vi "Init Package.vi"(7 "Logger":refnum<class "Logger.lvclass">, 8 "error in (no error)":errorcluster, 11 "GPackCLI in":refnum<class "GPackCLI.lvclass">) -> (0 "error out":errorcluster, 3 "GPackCLI out":refnum<class "GPackCLI.lvclass">)   [LabVIEW 2020, in "GPackTools.lvlib" / "GPackCLI.lvclass"]
uses:
  GPackCLI.lvclass
  GPack/Logger/Logger.lvclass
  GPackCLI.lvclass/GPackCLI.ctl
  CLIAction/CLIAction.lvclass
  GPack/PackageAbstract/PackageAbstract.lvclass
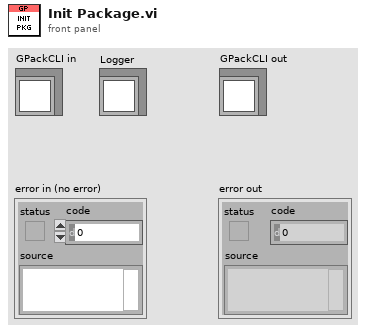
[diagram p1: front panel]
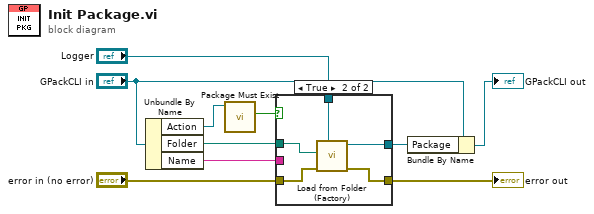
[diagram p0: block diagram]
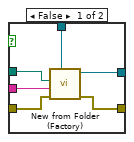
[diagram p2: hidden frame]
diagram:
  n1 = Unbundle By Name("GPackCLI in") -> ("Action"=w3:refnum<class "CLIAction.lvclass">, "Folder"=w9:path, "Name"=w6:string)
  n2 = call-dynamic "Package Must Exist.vi"("CLIAction in"=w3) -> ("Pkg Must Exist"=w2:bool)  [unwired: 8 in, 2 out]
  n3 = case shown="True" w2 {
    tunnel: w9 -> [w16 w21]
    tunnel: [w15 w20] -> w7
    tunnel: w6 -> [w14 _]
    tunnel: "error in (no error)" -> [w13 w19]
    tunnel: [w12 w18] -> w4
    tunnel: "Logger" -> [w11 w17]
    frame False {
      n4 = call "New from Folder (Factory).vi"("Logger"=w11, "error in (no error)"=w13, "Name (Auto)"=w14, "Folder"=w16) -> ("error out"=w12:errorcluster, "PackageAbstract out"=w15:refnum<class "PackageAbstract.lvclass">)  [unwired: 6 in]
    }
    frame True {
      n5 = call "Load from Folder (Factory).vi"("Logger"=w17, "error in (no error)"=w19, "Folder"=w21) -> ("error out"=w18:errorcluster, "PackageAbstract out"=w20:refnum<class "PackageAbstract.lvclass">)  [unwired: 7 in]
    }
  }
  "error out" <- w4
  n6 = Bundle By Name(cluster="GPackCLI in", "Package"=w7) -> (→"GPackCLI out":refnum<class "GPackCLI.lvclass">)
